vi "PDF_Interface_PDF Protokoll EPA1065_InterferenceVerification.vi"(8 "error in (no error)":errorcluster caption="Fehler (Eingang, kein Fehler)", 11 "Save PDF File Path":path) -> (0 "error out":errorcluster caption="Fehler (Ausgang)")   [LabVIEW 2020, in "EPA 1065.lvlib" / "Interference verificaton 1065-366.lvlib"]
uses:
  Interference verificaton 1065-366.lvlib
  Visualisierungs Elemente/String - Ausgabefeld.ctl
  ResultTable.ctl
  Sprachverwaltung/FGV Aktion Tabelle zerlegen.ctl
  <vilib>/Utility/miscctls.llb/LVRowAndColumnTypeDef.ctl
  Aktion FGV Interference.ctl
  Seiten/FT-IR/FGV FT-IR Aktionen.ctl
  Aktion Index uebersetzten.ctl
  Seiten/System Einstellungen V2/Aktioen FGV System Konstanten.ctl
  PDF_Interface/PDF Protokoll Standard Kopf Optionen.ctl
  <vilib>/Simplicity AI/SAI_PDF_API/Classes/Context/Controls/SAI_PDF_PDF Details.ctl
  PDF_Interface/PDF Interface Helper/PDFContentType.ctl
  PDF_Interface/PDF Interface Helper/PDFTableContentType.ctl
  PDF_Interface/PDF Interface Helper/PDFResults.ctl
  PDF_Interface/PDF Interface Helper/PDFResultPictures.ctl
  PDF_Interface/PDF Interface Helper/PDFCommentPosition.ctl
  PDF_Interface/PDF Interface Helper/PDFPageBreak.ctl
  PDF_Interface/PDF Interface Helper/PDFTablePictures.ctl
  PDF_Interface/PDF Interface Helper/PDFBemerkung.ctl
  <vilib>/Simplicity AI/SAI_PDF_API/Classes/Context/Controls/SAI_PDF_Text Align.ctl
  <vilib>/Simplicity AI/SAI_PDF_API/Classes/Context/Controls/SAI_PDF_Font.ctl
  <vilib>/Simplicity AI/SAI_PDF_API/Classes/Context/Controls/SAI_PDF_Font Encoding.ctl
  Allgemein/allgemeine Sub-VIs.lvlib
  Seiten/FT-IR/Span/Spanfaktor.lvlib
  Seiten/FT-IR/FT-IR.lvlib
  Sprachverwaltung/Sprachverwaltung.lvlib
  Seiten/System Einstellungen V2/System Einstellungen V2.lvlib
  PDF_Interface/PDF Interface.lvlib
  PDF_Interface/PDF Interface Helper/PDF Interface Helper.lvlib
  <vilib>/Simplicity AI/SAI_PDF_API/Classes/Context/Context.lvclass
  Linearisierung V2/Protokoll/Protokoll.lvlib
panel:
  out "Grenze in ppm:":sgl=2.0 caption="Limit in ppm:" min=0 format="%#.6g"
  out "[%]":sgl=2.0 caption="Limit:" min=0 format="%#.6g"
  out "LIN Ausgabetabelle":T1
  out "[%]":sgl=120.0 caption="Interference:" min=0 format="%#.6g"
  out "Konzentration Komponente":sgl=120.0 caption="Concentration:" min=0
  out "Komponente:":T2 caption="ppm"
  out "max. Flow Weighted Mean:":T2 caption="%"
  out "Konzentration FlowWeightedMean":sgl=120.0 caption="Concentration:" min=0 format="%#.2f"
  out "Ergebnis Tabelle":string[][](table) caption="Tabelle 3"
  out "Header Tabelle":string[][](table) caption="Tabelle"
  # "Interference Verification - EPA § 1065.366"
  # "Result"
  # "Analysis"
  # "Interference for Component:"
  # "Expected Flow weighted mean:"
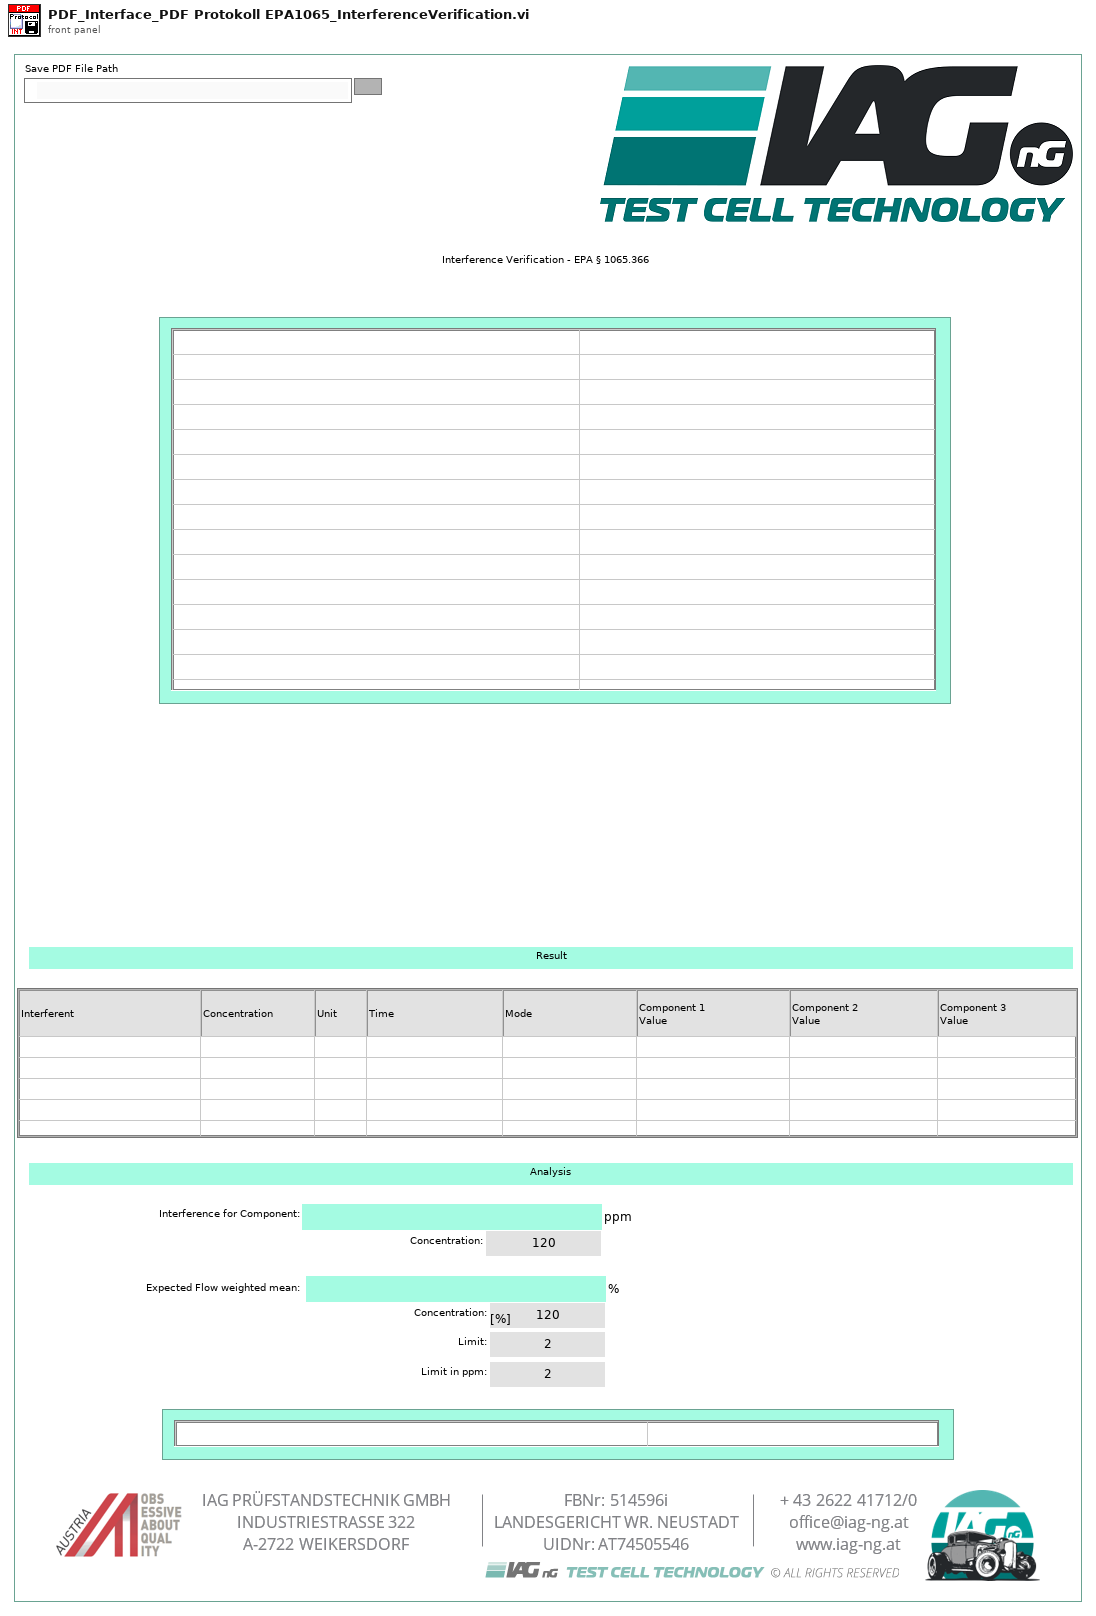
[diagram p1: front panel]
types:
  T1 = typedef "EPA 1065.lvlib/Interference verificaton 1065-366.lvlib/ResultTable.ctl" = string[][]
  T2 = typedef "String - Ausgabefeld.ctl" = string
  T3 = typedef "Sprachverwaltung.lvlib/FGV Aktion Tabelle zerlegen.ctl" = enum16{"laden", "vereinzeln", "speichern"}
  T4 = typedef "PDF Interface.lvlib/PDF Protokoll Standard Kopf Optionen.ctl" = cluster{"Analysator":bool, "FT-IR Rezept":bool, "Gasteiler":bool, "Gas Komponente":bool, "Gas Flasche":bool, "LIN Protokoll":bool, "Operator":bool}
  T5 = typedef "System Einstellungen V2.lvlib/Aktioen FGV System Konstanten.ctl" = enum16{"lesen", "laden", "speichern", "Sprache"}
  T6 = typedef "EPA 1065.lvlib/Interference verificaton 1065-366.lvlib/Aktion Index uebersetzten.ctl" = enum16{"lesen", "schreiben", "auswerten"}
  T7 = typedef "FT-IR.lvlib/FGV FT-IR Aktionen.ctl" = enum16{"lesen", "NOG setzen", "NOS setzen", "Initialisieren", "speichern", "ALLES setzen", "FT-IR Spektrum loggen", "Komm Stoppen", "Spektrum LogKonfig"}
  T8 = typedef "EPA 1065.lvlib/Interference verificaton 1065-366.lvlib/Aktion FGV Interference.ctl" = enum16{"Lesen", "TestKonfig", "TestSetting", "Einheiten", "Ergebnis", "Laden", "Tabelle", "Speichern", "löschen"}
  T9 = typedef "LVRowAndColumnTypeDef.ctl" = cluster{"Row":i32, "Column":i32}
  T10 = typedef "PDF Interface.lvlib/PDF Interface Helper.lvlib/PDFPageBreak.ctl" = enum16{"none", "before", "after", "after comment"}
  T11 = typedef "PDF Interface.lvlib/PDF Interface Helper.lvlib/PDFResults.ctl" = cluster{"Results":cluster{"Result Text":string, "Result":bool}[], "ResultPictures":T12, "use Pictures":bool, "Image Scale (%)":sgl, "Autoscale? (T)":bool, "Horizontal Align":i32, "Position":i32}
  T12 = typedef "PDF Interface.lvlib/PDF Interface Helper.lvlib/PDFResultPictures.ctl" = cluster{"Yes Ctl Refnum":refnum<vi>, "No Ctl Refnum":refnum<vi>}
  T13 = typedef "PDF Interface.lvlib/PDF Interface Helper.lvlib/PDFContentType.ctl" = cluster{"Titel":string, "Header Table":string[][], "Table Array":T14[], "Bemerkungen":T17[]}
  T14 = typedef "PDF Interface.lvlib/PDF Interface Helper.lvlib/PDFTableContentType.ctl" = cluster{"TableHeader":string[], "Table":string[][], "Relative Column Widths (%)":sgl[], "Results":T11, "PositionBemerkung":T15, "PageBreak":T10, "TablePictures":T16, "Horizontal Align":i32}
  T15 = typedef "PDF Interface.lvlib/PDF Interface Helper.lvlib/PDFCommentPosition.ctl" = enum16{"before", "after"}
  T16 = typedef "PDF Interface.lvlib/PDF Interface Helper.lvlib/PDFTablePictures.ctl" = cluster{"Ctl Refnum In":refnum<vi>[], "RowOrColumn":enum16{"Row", "Column"}, "IndexToInsert":u16, "Image Scale (%)":sgl[], "Autoscale? (T)":bool[], "Horizontal Align":i32}
  T17 = typedef "PDF Interface.lvlib/PDF Interface Helper.lvlib/PDFBemerkung.ctl" = cluster{"Bemerkung Text":string, "Align (Left)":T18, "Add Line Feeds (F:No)":bool, "Font":T19}
  T18 = typedef "SAI_PDF_Toolkit.lvlib/Context.lvclass/SAI_PDF_Text Align.ctl" = i32
  T19 = typedef "SAI_PDF_Toolkit.lvlib/Context.lvclass/SAI_PDF_Font.ctl" = cluster{"Font":string, "Size":i32, "Colour":u32, "Bold":bool, "Italic":bool, "Underline":bool, "Strikethrough":bool, "Font Encoding":T20}
  T20 = typedef "SAI_PDF_Toolkit.lvlib/Context.lvclass/SAI_PDF_Font Encoding.ctl" = enum16{"Cp1252, WinANSI", "IdentityH", "IdentityV", "Cp1250", "Cp1257", "MacRoman"}
  T21 = typedef "SAI_PDF_Toolkit.lvlib/Context.lvclass/SAI_PDF_PDF Details.ctl" = cluster{"Title":string, "Subject":string, "Keywords":string, "Author":string, "Creator":string}
  T22 = cluster{"Header Footer Text Cluster":cluster{"Header Text":string, "Footer Text":string, "Time":string, "Page Number":string}, "PDF Details":T21}
  T23 = typedef "EPA 1065.lvlib/Interference verificaton 1065-366.lvlib/TestSetting.ctl" = cluster{"Bearbeiter:":string, "Pfad:":path, "Textname:":string, "Analysator":T24}
  T24 = typedef "System Einstellungen V2.lvlib/Analysatoren.ctl" = string
  T25 = typedef "EPA 1065.lvlib/Interference verificaton 1065-366.lvlib/TestKonfig.ctl" = cluster{"CH4:":u16, "Ethane:":u16, "NMHC:":u16, "NMNEHC:":u16, "Komp 1 aktiv:":bool, "Komp 2 aktiv:":bool, "Komp 3 aktiv:":bool, "Komp 4 aktiv:":bool, "Modus":T26, "CG Aufschaltzeit:":dbl, "Interferent 1: CO2":u16, "Interferent 2: H2O":u16, "Interferent 3: CH4":u16, "Interferent 4: C2H6 / C3H8":u16, "Gasflaschen Nr.:":string, "Gasflaschen Nr.: 3":string, "Gasflaschen Nr.: 4":string, "Inter 1 aktiv":bool, "Inter 2 aktiv":bool, "Inter 3 aktiv":bool, "Inter 4 aktiv":bool, "Accuracy":string, "Accuracy 3":string, "Accuracy 4":string, "Konzentration 1:":dbl, "Konzentration 2:":dbl, "Konzentration 3:":dbl, "Konzentration 4:":dbl, "Flow weighted mean 1:":dbl, "Flow weighted mean 2:":dbl, "Flow weighted mean 3:":dbl, "Flow weighted mean 4:":dbl}
  T26 = typedef "EPA 1065.lvlib/Interference verificaton 1065-366.lvlib/Modus.ctl" = u16
  T27 = typedef "EPA 1065.lvlib/Interference verificaton 1065-366.lvlib/Komponenten.ctl" = cluster{"Komponente":T2, "Komponente Index":i32, "Komponente 2":T2, "Komponente Index 2":i32, "Komponente 3":T2, "Komponente Index 3":i32, "Komponente 4":T2, "Komponente Index 4":i32, "Interferent 1":T2, "Interferent Index":i32, "Interferent 2":T2, "Interferent 2 Index":i32, "Interferent 3":T2, "Interferent 3 Index":i32, "Interferent 4":T2, "Interferent 4 Index":i32}
  T28 = cluster{"Modell":string, "ProjektNummer":string, "Software Version":string, "Seriennummer":string}
  T29 = cluster{"Header Size":i32, "Column Ratio left":sgl[]}
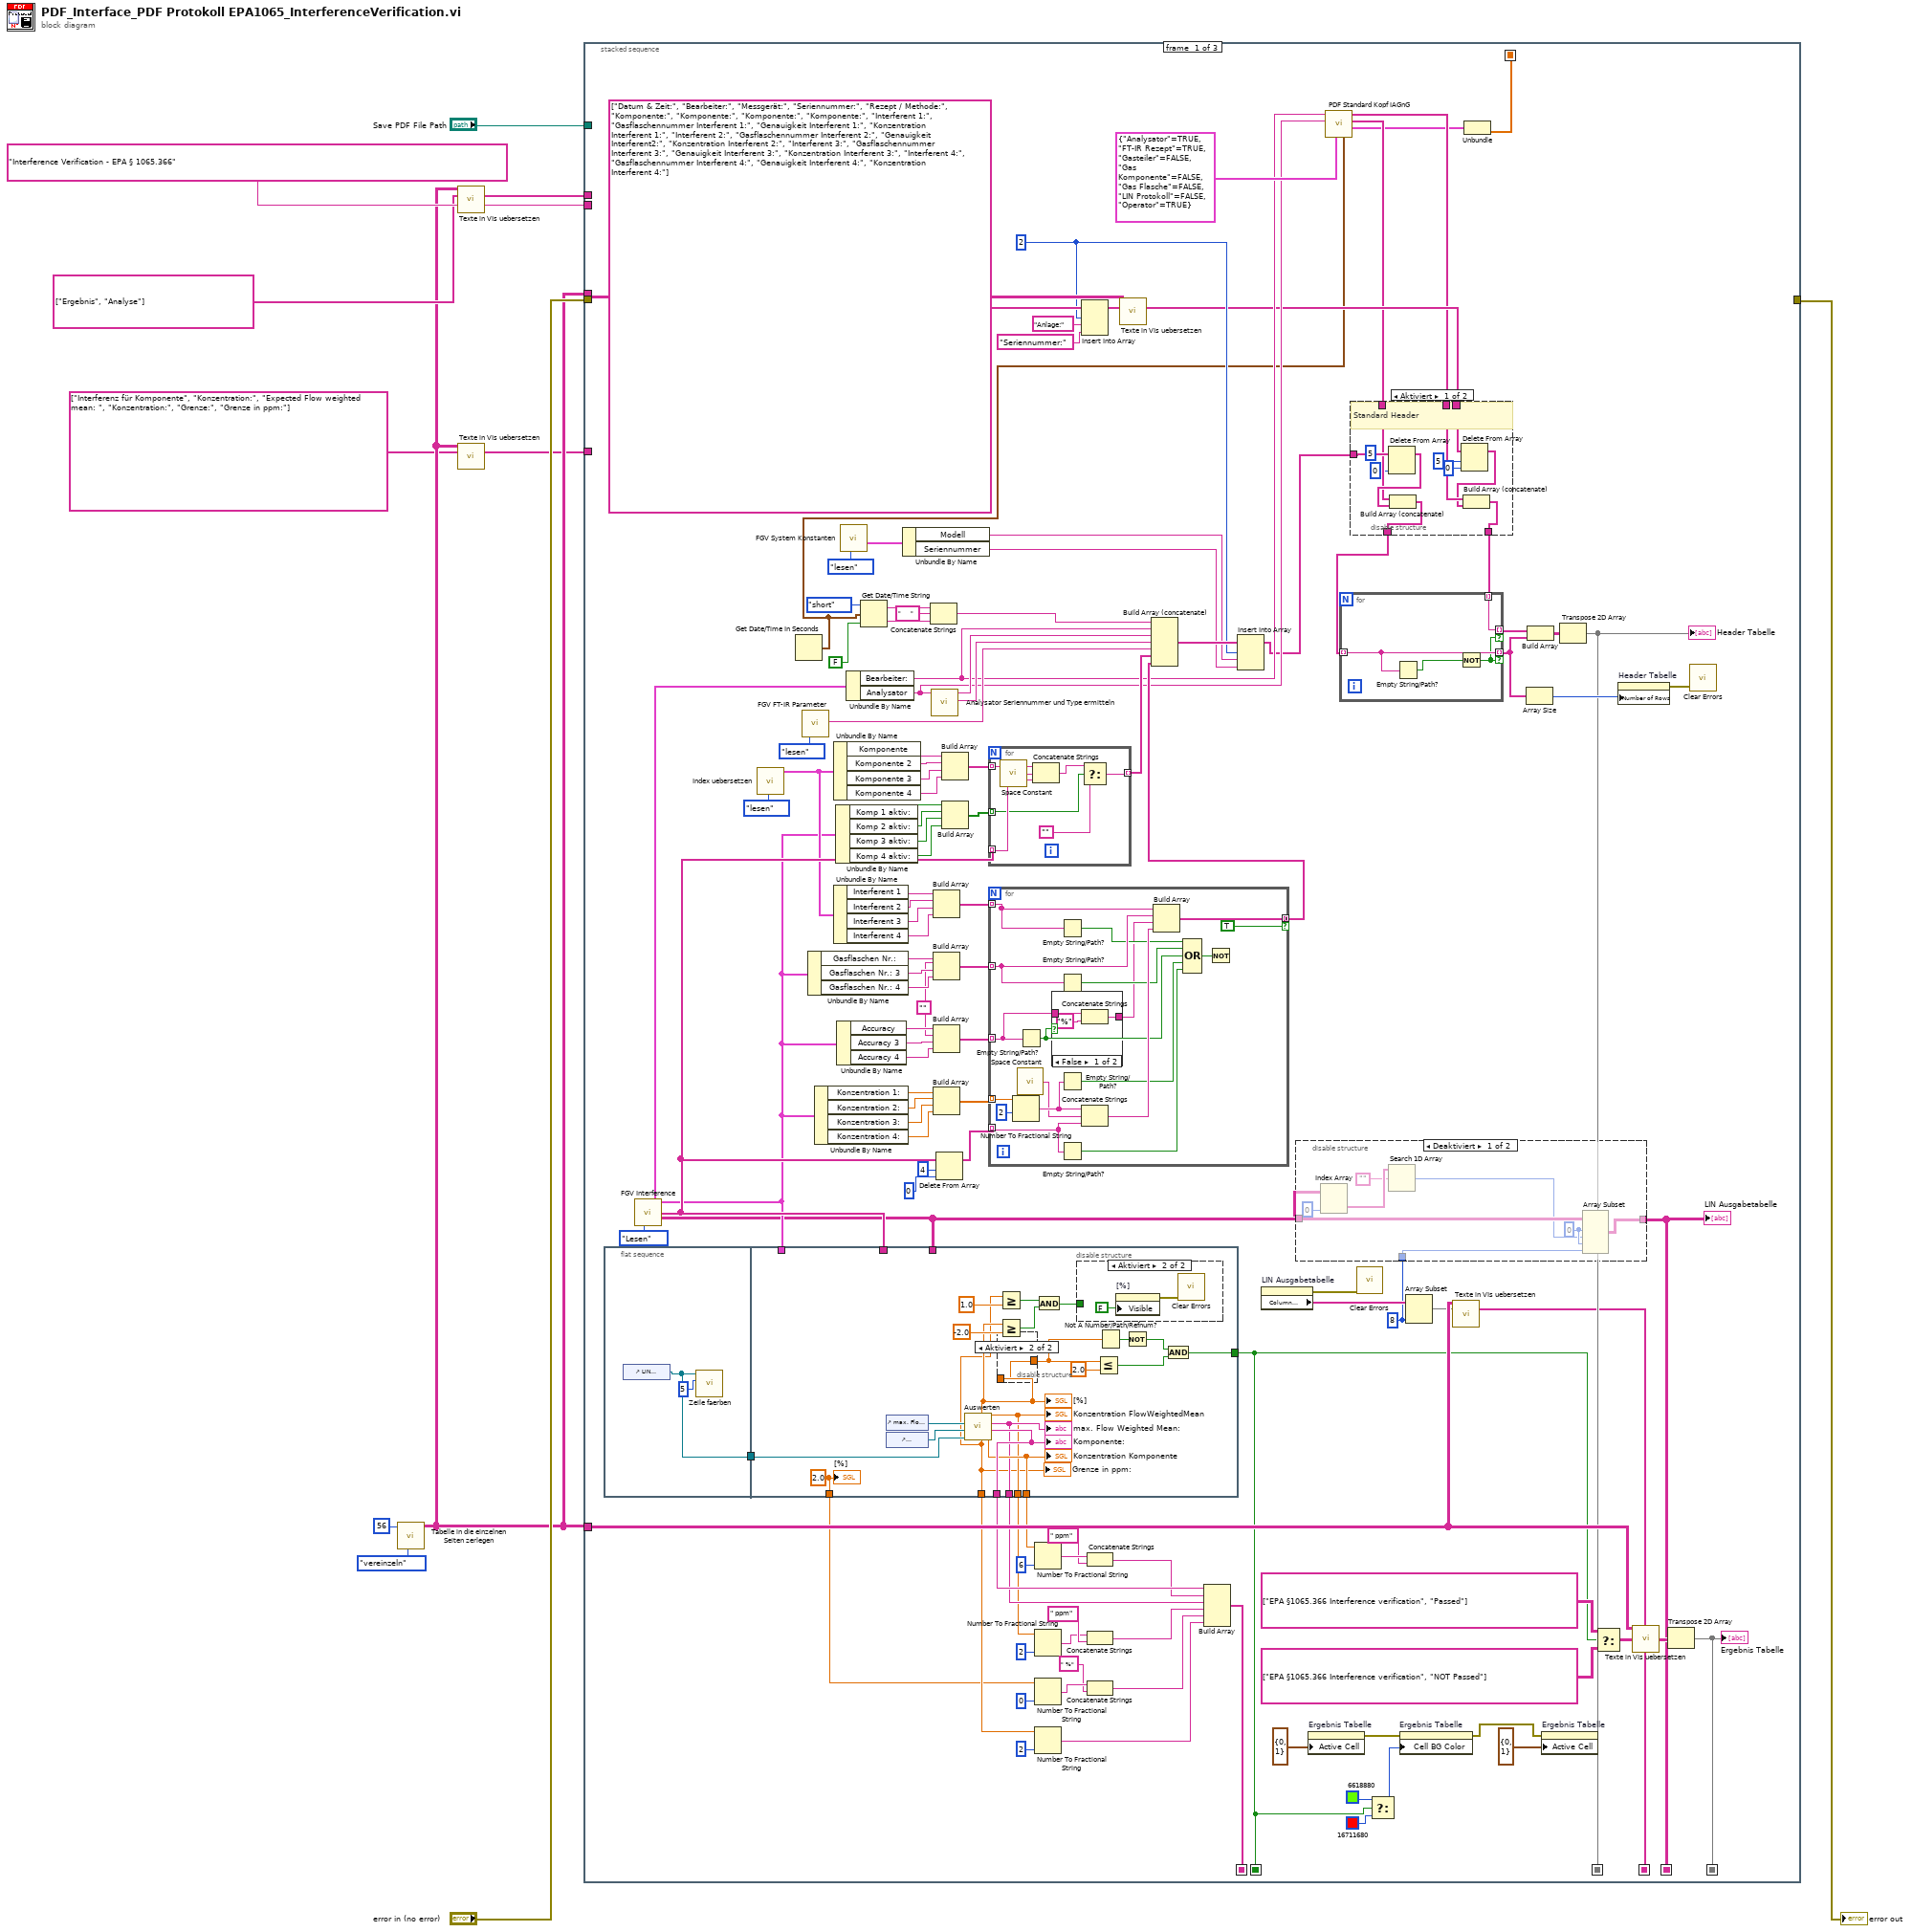
[diagram p0: block diagram]
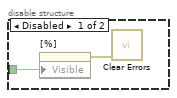
[diagram p5: hidden frame]
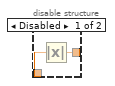
[diagram p6: hidden frame]
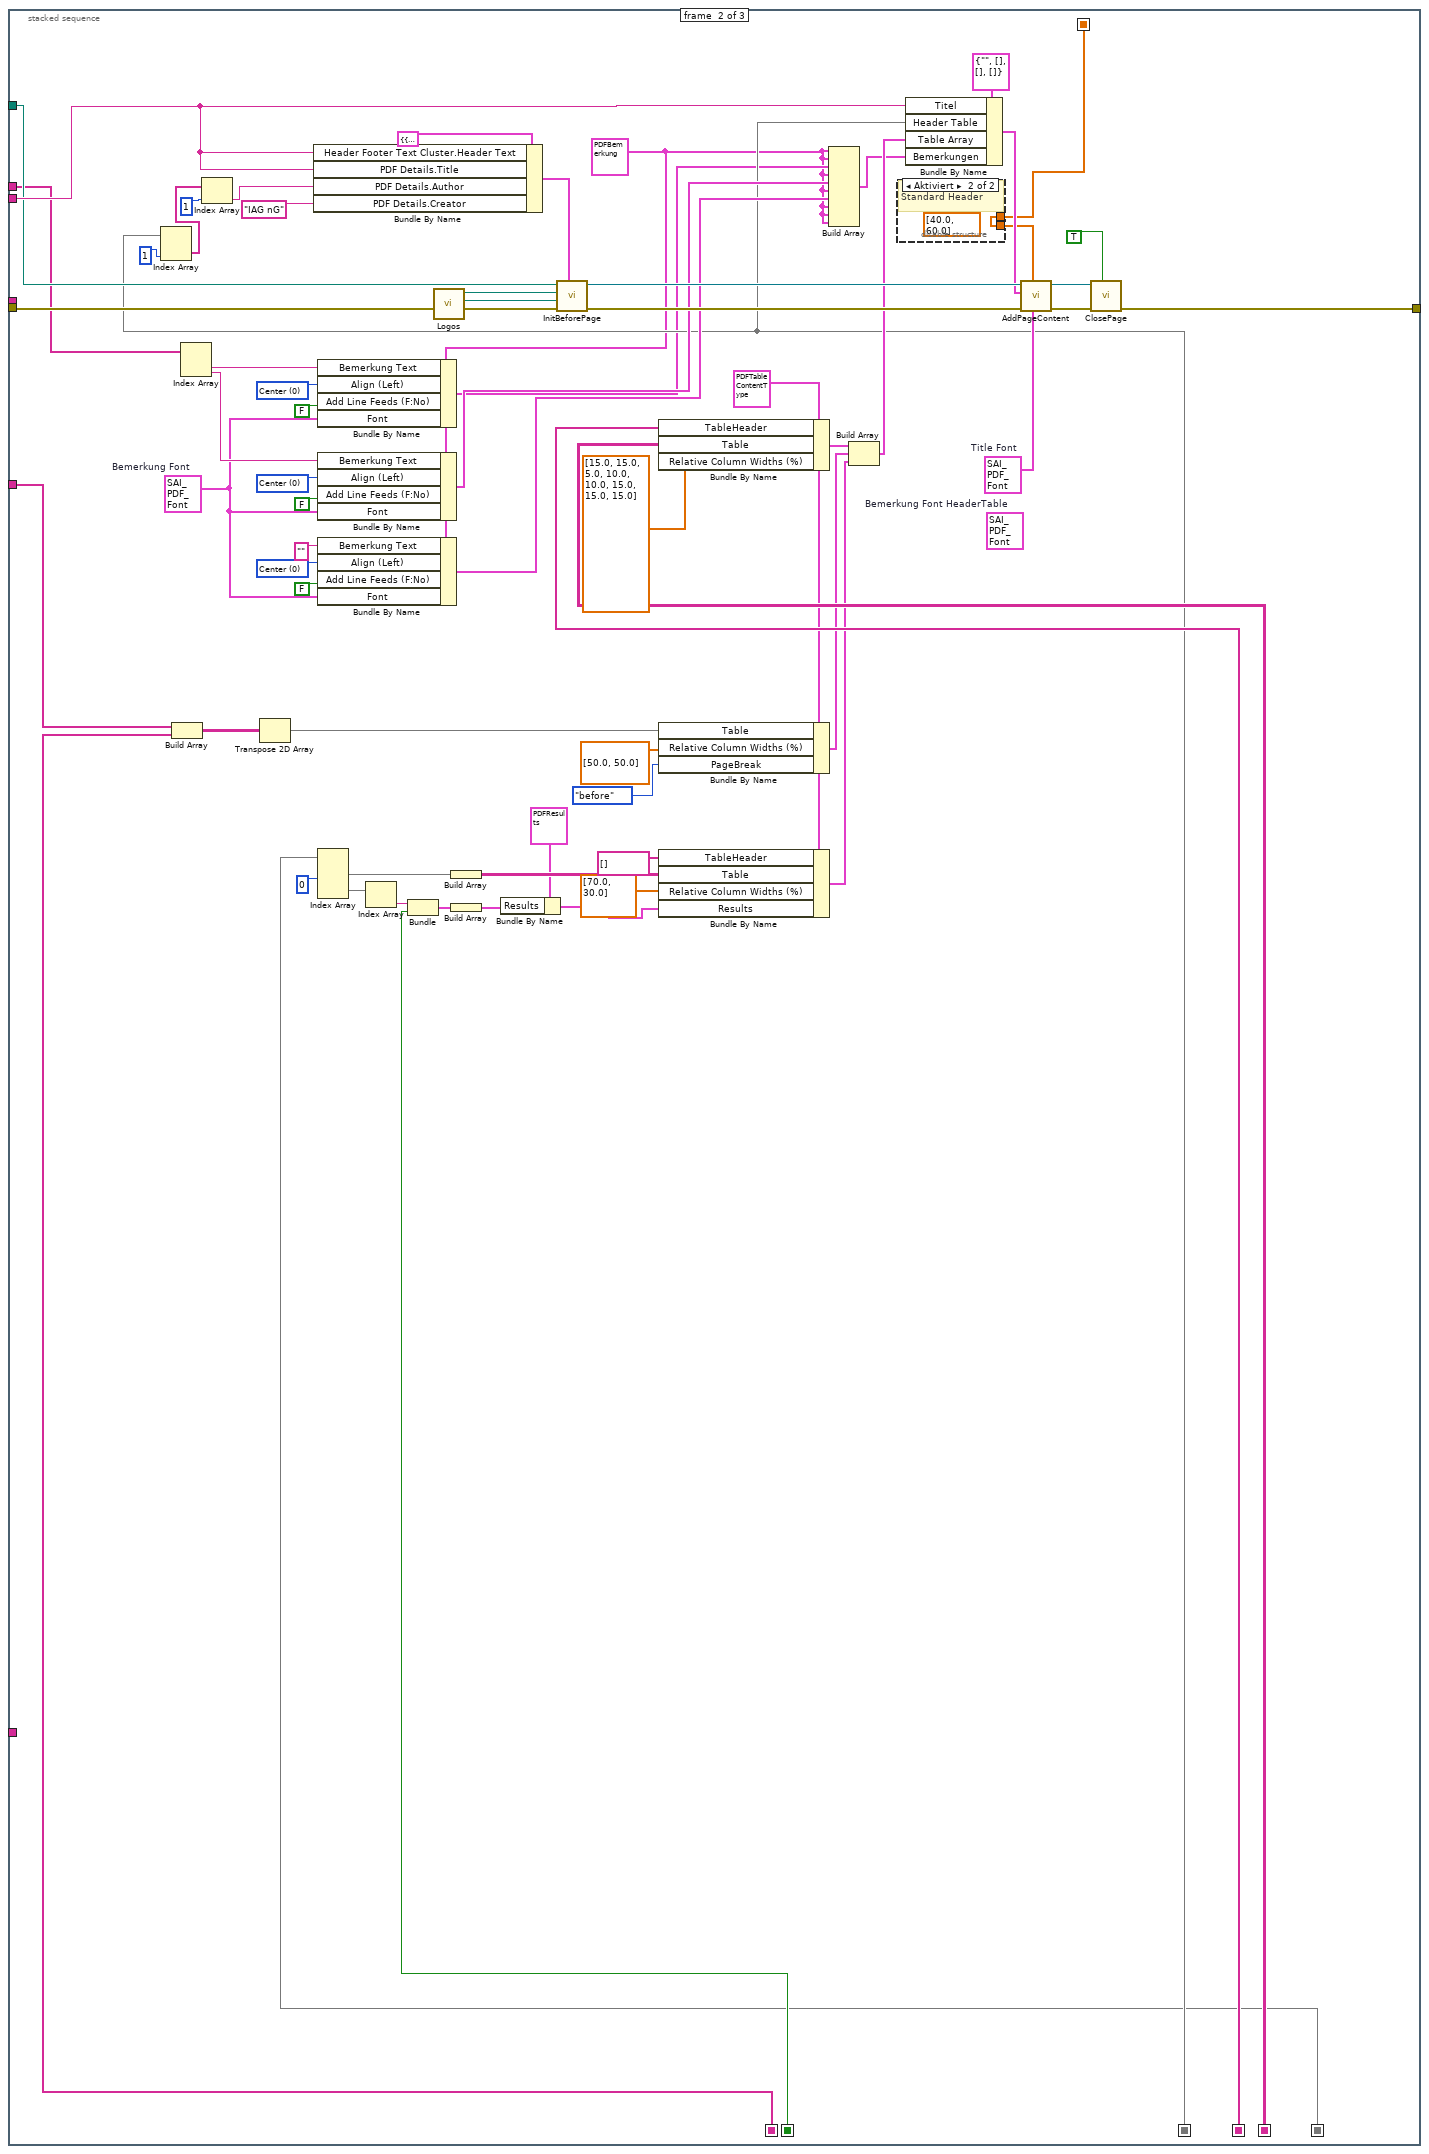
[diagram p7: hidden frame]
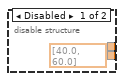
[diagram p8: hidden frame]
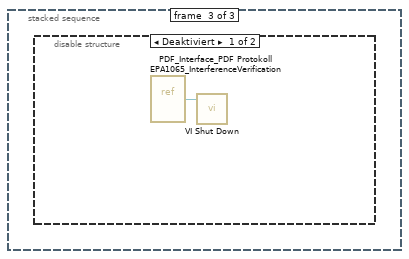
[diagram p9: hidden frame]
diagram:
  n1 = call "Tabelle in die einzelnen Seiten zerlegen.vi"("Aktion"=FGV_Aktion_Tabelle_zerlegen."vereinzeln", "Index (Seite)"=56) -> ("Sprachliste"=w3:string[][])  [unwired: 7 in, 2 out]
  n2 = call "Texte in VIs uebersetzen.vi"("Sprachliste"=w3, "String-Array zum Übersetzen"=string[] ["Ergebnis", "Analyse"], "String zum Übersetzen"="Interference Verification - EPA § 1065.366") -> ("String-Array zum Übersetzen"=w7:string[], "String zum Übersetzen"=w6:string)  [unwired: 8 in, 3 out]
  n3 = call "Texte in VIs uebersetzen.vi"("Sprachliste"=w3, "String-Array zum Übersetzen"=string[] ["Interferenz für Komponente", "Konzentration:", "Expected Flow weighted mean: ", "Konzentration:", "Grenze:", "Grenze in ppm:"]) -> ("String-Array zum Übersetzen"=w1:string[])  [unwired: 9 in, 4 out]
  n4 = stacked-sequence {
    seq-local: [w56 _ _] -> [_ w243 _]
    seq-local: [w55 _ _] -> [_ w244 _]
    seq-local: [w57 _ _] -> [_ w254 _]
    seq-local: [w37 _ _] -> [_ w249 _]
    seq-local: [w31 _ _] -> [_ w264 _]
    seq-local: [w36 _ _] -> [_ w265 _]
    seq-local: [w13 _ _] -> [_ w221 _]
    tunnel: w3 -> [w58 _ _]
    tunnel: w3 -> [w72 _ _]
    tunnel: "Save PDF File Path" -> [_ w268 _]
    tunnel: w7 -> [_ w255 _]
    tunnel: w6 -> [_ w269 _]
    tunnel: "error in (no error)" -> [_ w267 _]
    tunnel: [_ w266 _] -> w4
    tunnel: w1 -> [_ w230 _]
    frame #0 {
      w32 = 8 ("Länge")
      w61 = ""
      w62 = 2 ("Index")
      n5 = flat-sequence {
        tunnel: [w191] -> w125
        tunnel: w125 -> [w213]
        tunnel: [w205] -> w55
        tunnel: w99 -> [_]
        tunnel: w30 -> [_]
        tunnel: w71 -> [_]
        tunnel: [w198] -> w54
        tunnel: [w197] -> w53
        tunnel: [w196] -> w48
        tunnel: [w195] -> w46
        tunnel: [w194] -> w41
        tunnel: [w193] -> w38
        frame #0 {
          n6 = control-ref of="LIN Ausgabetabelle"() -> (w191:refnum<vi>)
          n7 = call "Zeile faerben.vi"("Anzahl"=5, "Table (Eingang)"=w191) -> ()  [unwired: 9 in, 1 out]
        }
        frame #1 {
          w193 = sgl 2.0 ("[%]")
          n8 = control-ref of="max. Flow Weighted Mean:"() -> (w212:refnum<vi>)
          n9 = control-ref of="Komponente:"() -> (w211:refnum<vi>)
          n10 = call "Auswerten.vi"("LIN Ausgabetabelle"=w213, "Komponente:"=w211, "max. Flow Weighted Mean:"=w212) -> ("Konzentration Komponente"=w197:dbl, "Komponente:"=w198:T2, "max. Flow Weighted Mean:"=w196:T2, "Konzentration FlowWeightedMean"=w195:dbl, "Limit in ppm"=w194:dbl, "[%]"=w200:dbl)  [unwired: 3 in]
          "max. Flow Weighted Mean:" <- w196
          "Konzentration FlowWeightedMean" <- w195
          "Konzentration Komponente" <- w197
          "Komponente:" <- w198
          "[%]" <- w200
          "Grenze in ppm:" <- w194
          n11 = disable-structure shown="Aktiviert" {
            disable-tunnel: w200 -> [w219 w220]
            disable-tunnel: [w218 w220] -> w209
            frame Disabled {
              n12 = Absolute Value(x=w219) -> (abs(x)=w218:dbl)
            }
            frame Enabled {
            }
          }
          n13 = Greater Or Equal?(x=w194, y=1.0) -> (x >= y?=w202:bool)
          n14 = Greater Or Equal?(x=w200, y=-2.0) -> (x >= y?=w201:bool)
          n15 = And(x=w202, y=w201) -> (x .and. y?=w199:bool)
          n16 = disable-structure shown="Aktiviert" {
            disable-tunnel: w199 -> [w215 _]
            frame Disabled {
              n17 = property on="[%]" class="DigWert (strikt)"("Visible"=w215) -> (error out=w214:errorcluster)  [unwired: 2 in, 1 out]
              n18 = call <vilib>:"Clear Errors.vi"("error in (no error)"=w214) -> ()  [unwired: 5 in, 2 out]
            }
            frame Enabled {
              n19 = property on="[%]" class="DigWert (strikt)"("Visible"=FALSE ("Sichtbar")) -> (error out=w217:errorcluster)  [unwired: 2 in, 1 out]
              n20 = call <vilib>:"Clear Errors.vi"("error in (no error)"=w217) -> ()  [unwired: 5 in, 2 out]
            }
          }
          n21 = Less Or Equal?(x=w209, y=2.0) -> (x <= y?=w207:bool)
          n22 = Not A Number/Path/Refnum?(number/path/refnum=w209) -> (NaN/Path/Refnum?=w208:bool)
          n23 = Not(x=w208) -> (.not. x?=w206:bool)
          n24 = And(x=w206, y=w207) -> (x .and. y?=w205:bool)
          "[%]" <- w193
        }
      }
      n25 = call "FGV Interference.vi"("Aktion FGV Interference"=Aktion_FGV_Interference."Lesen") -> ("TestSetting"=w123:T23, "TestKonfig"=w71:T25, "Êinheiten"=w99:string[], "Tabelle"=w30:T2[][])  [unwired: 9 in, 2 out]
      n26 = call "Index uebersetzen.vi"("Aktion"=Aktion_Index_uebersetzten."lesen") -> ("Komponenten"=w93:T27)  [unwired: 9 in, 1 out]
      n27 = Get Date/Time In Seconds() -> (seconds since 1Jan1904=w18:timestamp)
      n28 = call "FGV FT-IR Parameter.vi"("Aktion"=FGV_FT-IR_Aktionen."lesen") -> ("Current Recipe"=w105:string)  [unwired: 11 in, 7 out]
      n29 = Unbundle By Name(w71) -> ("Gasflaschen Nr.:"=w92:string, "Gasflaschen Nr.: 3"=w91:string, "Gasflaschen Nr.: 4"=w90:string)
      n30 = Unbundle By Name(w71) -> ("Konzentration 1:"=w89:dbl, "Konzentration 2:"=w88:dbl, "Konzentration 3:"=w87:dbl, "Konzentration 4:"=w86:dbl)
      n31 = Unbundle By Name(w93) -> ("Komponente"=w115:T2, "Komponente 2"=w114:T2, "Komponente 3"=w113:T2, "Komponente 4"=w60:T2)
      n32 = Unbundle By Name(w93) -> ("Interferent 1"=w97:T2, "Interferent 2"=w96:T2, "Interferent 3"=w95:T2, "Interferent 4"=w94:T2)
      n33 = Unbundle By Name(w71) -> ("Komp 1 aktiv:"=w112:bool, "Komp 2 aktiv:"=w111:bool, "Komp 3 aktiv:"=w110:bool, "Komp 4 aktiv:"=w59:bool)
      n34 = Unbundle By Name(w71) -> ("Accuracy"=w79:string, "Accuracy 3"=w78:string, "Accuracy 4"=w77:string)
      n35 = call "FGV System Konstanten.vi"("Aktionen"=Aktioen_FGV_System_Konstanten."lesen") -> ("Cluster out"=w69:T28)  [unwired: 6 in, 4 out]
      n36 = Unbundle By Name(w123) -> ("Bearbeiter:"=w26:string, "Analysator"=w25:T24)
      n37 = Get Date/Time String(date format (0)=enum16{"short", "long", "abbreviated"}."short" ("Datumsformat (0)"), seconds (now)=w18, want seconds? (F)=FALSE ("Angabe von Sekunden? (F)")) -> (date string=w122:string, time string=w121:string)
      n38 = Unbundle By Name(w69) -> ("Modell"=w66:string, "Seriennummer"=w65:string)
      n39 = Concatenate Strings(w122, "     " ("String"), w121) -> (w107:string)
      n40 = call "Analysator Seriennummer und Type ermitteln.vi"("Analysator"=w25) -> ("Type"=w28:string, "Name für Protokoll"=w29:string)  [unwired: 8 in, 1 out]
      n41 = Build Array(w97, w96, w95, w94) -> (w85:T2[])
      n42 = Build Array(w92, w61, w91, w90) -> (w84:string[])
      n43 = Build Array(w79, w61, w78, w77) -> (w76:string[])
      n44 = Build Array(w89, w88, w87, w86) -> (w83:dbl[])
      n45 = Delete From Array(array=w99, length=4 ("Länge"), index=0 ("Index")) -> (array with subset deleted=w81:string[])  [unwired: 1 out]
      n46 = Build Array(w115, w114, w113, w60) -> (w109:T2[])
      n47 = Build Array(w112, w111, w110, w59) -> (w108:bool[])
      n48 = for {
        tunnel: [w187] -> w106 mode=indexing
        tunnel: w109 -> [w190] mode=indexing
        tunnel: w108 -> [w186] mode=indexing
        tunnel: w99 -> [w189] mode=indexing
        n49 = call <vilib>:"Space Constant.vi"() -> ("String"=w188:string)
        n50 = Concatenate Strings(w190, w188, w189) -> (w185:string)
        n51 = Select(t=w185, s=w186, f="") -> (s? t:f=w187:string)
      }
      n52 = for {
        tunnel: w85 -> [w172] mode=indexing
        tunnel: w84 -> [w171] mode=indexing
        tunnel: w83 -> [w175] mode=indexing
        tunnel: w81 -> [w174] mode=indexing
        tunnel: [w169] -> w80 mode=concatenating if=TRUE
        tunnel: w76 -> [w159] mode=indexing
        n53 = Number To Fractional String(number=w175, precision (6)=i16 2 ("Genauigkeit (6)")) -> (F-format string=w173:string)  [unwired: 2 in]
        n54 = call <vilib>:"Space Constant.vi"() -> ("String"=w163:string)
        n55 = Empty String/Path?(string/path=w159) -> (empty?=w158:bool)
        n56 = case shown="False" w158 {
          tunnel: [w177 w179] -> w162
          tunnel: w159 -> [w176 w179]
          frame False {
            n57 = Concatenate Strings(w176, "%" ("String")) -> (w177:string)
          }
          frame True {
          }
        }
        n58 = Empty String/Path?(string/path=w172) -> (empty?=w168:bool)
        n59 = Empty String/Path?(string/path=w171) -> (empty?=w167:bool)
        n60 = Empty String/Path?(string/path=w173) -> (empty?=w164:bool)
        n61 = Empty String/Path?(string/path=w174) -> (empty?=w166:bool)
        n62 = Concatenate Strings(w173, w163, w174) -> (w170:string)
        n63 = Build Array(w172, w171, w162, w170) -> (w169:T2[])
        n64 = Compound Arithmetic op=OR ("Mehrfacharithmetik")(w168, w167, w158, w164, w166) -> (w165:bool)
        n65 = Not(x=w165) -> ()  [unwired: 1 out]
      }
      n66 = Number To Fractional String(number=w53, precision (6)=i16 6 ("Genauigkeit (6)")) -> (F-format string=w51:string)  [unwired: 2 in]
      n67 = Number To Fractional String(number=w46, precision (6)=i16 2 ("Genauigkeit (6)")) -> (F-format string=w44:string)  [unwired: 2 in]
      n68 = Number To Fractional String(number=w38, precision (6)=i16 0 ("Genauigkeit (6)")) -> (F-format string=w17:string)  [unwired: 2 in]
      n69 = Number To Fractional String(number=w41, precision (6)=i16 2 ("Genauigkeit (6)")) -> (F-format string=w40:string)  [unwired: 2 in]
      n70 = Insert Into Array(array=string[] ["Datum & Zeit:", "Bearbeiter:", "Messgerät:", "Seriennummer:", "Rezept / Methode:", "Komponente:", "Komponente:", "Komponente:", "Komponente:", "Interferent 1:", "Gasflaschennummer Interferent 1:", "Genauigkeit Interferent 1:", "Konzentration Interferent 1:", "Interferent 2:", "Gasflaschennummer Interferent 2:", "Genauigkeit Interferent2:", "Konzentration Interferent 2:", "Interferent 3:", "Gasflaschennummer Interferent 3:", "Genauigkeit Interferent 3:", "Konzentration Interferent 3:", "Interferent 4:", "Gasflaschennummer Interferent 4:", "Genauigkeit Interferent 4:", "Konzentration Interferent 4:"], index=w62, new element #1="Anlage:" ("Neues Element/Teil-Array"), new element #2="Seriennummer:" ("Neues Element/Teil-Array")) -> (w68:string[])
      n71 = Concatenate Strings(w51, " ppm" ("String")) -> (w49:string)
      n72 = Concatenate Strings(w44, " ppm" ("String")) -> (w43:string)
      n73 = Concatenate Strings(w17, " %" ("String")) -> (w15:string)
      n74 = call "Texte in VIs uebersetzen.vi"("Sprachliste"=w72, "String-Array zum Übersetzen"=w68) -> ("String-Array zum Übersetzen"=w23:string[])  [unwired: 9 in, 4 out]
      n75 = Build Array (concatenate)(w107, w26, w29, w28, w105, w106, w80) -> (w67:T2[])
      n76 = Build Array(w54, w49, w48, w43, w15, w40) -> (w37:T2[])
      n77 = Insert Into Array(array=w67, index=w62, new element #1=w66, new element #2=w65) -> (w21:T2[])
      n78 = property on="LIN Ausgabetabelle" class="Tbl (strikt)"() -> (error out=w33:errorcluster, "Column Headers[]"=w35:string[])  [unwired: 2 in, 1 out]
      n79 = disable-structure shown="Deaktiviert" {
        disable-tunnel: w32 -> [w141 _]
        disable-tunnel: [w140 w143] -> w31
        disable-tunnel: w30 -> [w139 w143]
        frame Disabled {
          w142 = 0 ("Index")
          n80 = Index Array(array=w139, index (col)=0 ("Deaktivierter Index (Spalte)")) -> (element=w137:T2[])  [unwired: 1 in]
          n81 = Search 1D Array(1D array=w137, element="") -> (index of element=w135:i32)  [unwired: 1 in]
          n82 = Array Subset(array=w139, index (row)=w142, length (row)=w135, index (col)=w142, length (col)=w141) -> (w140:T2[][])
        }
        frame Enabled {
        }
      }
      "LIN Ausgabetabelle" <- w31
      n83 = property on="Ergebnis Tabelle" class="Tbl (strikt)"("Active Cell"=T9 {"Row"=0, "Column"=1} ("Aktive Zelle:Aktive Zelle")) -> (error out=w130:errorcluster)  [unwired: 2 in, 1 out]
      n84 = call "PDF Standard Kopf IAGnG.vi"("Zeitstempel"=w18, "Oprtionen Cluster"=T4 {"Analysator"=TRUE, "FT-IR Rezept"=TRUE, "Gasteiler"=FALSE, "Gas Komponente"=FALSE, "Gas Flasche"=FALSE, "LIN Protokoll"=FALSE, "Operator"=TRUE}, "Analysator"=w25, "Bearbeiter/in"=w26) -> ("Size Cluster"=w14:T29, "Header Values"=w19:T2[], "Header Labels"=w22:string[])  [unwired: 4 in, 1 out]
      n85 = disable-structure shown="Aktiviert" {
        disable-tunnel: [w153 w157] -> w24
        disable-tunnel: w23 -> [w155 w157]
        disable-tunnel: w22 -> [w154 _]
        disable-tunnel: w21 -> [w149 w156]
        disable-tunnel: [w146 w156] -> w20
        disable-tunnel: w19 -> [w147 _]
        frame Enabled {
          # "Standard Header"
          n86 = Delete From Array(array=w149, length=5 ("Länge"), index=0 ("Index")) -> (array with subset deleted=w148:T2[])  [unwired: 1 out]
          n87 = Build Array (concatenate)(w147, w148) -> (w146:T2[])
          n88 = Delete From Array(array=w155, length=5 ("Länge"), index=0 ("Index")) -> (array with subset deleted=w152:string[])  [unwired: 1 out]
          n89 = Build Array (concatenate)(w154, w152) -> (w153:string[])
        }
        frame Disabled {
        }
      }
      n90 = for {
        tunnel: w20 -> [w183] mode=indexing
        tunnel: [w183] -> w102 mode=indexing if=w180
        tunnel: [w181] -> w104 mode=indexing if=w180
        tunnel: w24 -> [w181] mode=indexing
        n91 = Empty String/Path?(string/path=w183) -> (empty?=w182:bool)
        n92 = Not(x=w182) -> (.not. x?=w180:bool)
      }
      n93 = call <vilib>:"Clear Errors.vi"("error in (no error)"=w33) -> ()  [unwired: 5 in, 2 out]
      n94 = Select(t=u32 6618880, s=w55, f=u32 16711680) -> (s? t:f=w131:u32)
      n95 = property on="Ergebnis Tabelle" class="Tbl (strikt)"(error in=w130, "Cell BG Color"=w131) -> (error out=w126:errorcluster)  [unwired: 1 in, 1 out]
      n96 = Array Subset(array=w35, length=w32) -> (w34:string[])  [unwired: 1 in]
      n97 = call "Texte in VIs uebersetzen.vi"("Sprachliste"=w58, "String-Array zum Übersetzen"=w34) -> ("String-Array zum Übersetzen"=w36:string[])  [unwired: 9 in, 4 out]
      n98 = Unbundle(w14) -> ("Column Ratio left"=w13:sgl[])  [unwired: 1 out]
      n99 = Array Size(array=w102) -> (size(s)=w101:i32)
      n100 = Build Array(w104, w102) -> (w103:T2[][])
      n101 = property on="Ergebnis Tabelle" class="Tbl (strikt)"(error in=w126, "Active Cell"=T9 {"Row"=0, "Column"=1} ("Aktive Zelle:Aktive Zelle")) -> ()  [unwired: 1 in, 2 out]
      n102 = Transpose 2D Array(2D array=w103) -> (transposed array=w57:T2[][])
      "Header Tabelle" <- w57
      n103 = Select(t=string[][] [["EPA §1065.366 Interference verification"], ["Passed"]] ("Tabelle 3"), s=w55, f=string[][] [["EPA §1065.366 Interference verification"], ["NOT Passed"]] ("Tabelle 3")) -> (s? t:f=w75:string[][])
      n104 = property on="Header Tabelle" class="Tbl (strikt)"("Number of Rows"=w101) -> (error out=w100:errorcluster)  [unwired: 2 in, 1 out]
      n105 = call "Texte in VIs uebersetzen.vi"("Sprachliste"=w58, "2D String-Array zum Übersetzen"=w75) -> ("2D String-Array zum Übersetzen"=w74:string[][])  [unwired: 9 in, 4 out]
      n106 = Transpose 2D Array(2D array=w74) -> (transposed array=w56:string[][])
      "Ergebnis Tabelle" <- w56
      n107 = call <vilib>:"Clear Errors.vi"("error in (no error)"=w100) -> ()  [unwired: 5 in, 2 out]
    }
    frame #1 {
      w223 = T19 {"Font"="Arial", "Size"=12, "Colour"=0, "Bold"=TRUE, "Italic"=TRUE, "Underline"=FALSE, "Strikethrough"=FALSE, "Font Encoding"=enum."Cp1252, WinANSI"}  # Bemerkung Font
      w224 = T17 {"Bemerkung Text"="", "Align (Left)"=0, "Add Line Feeds (F:No)"=FALSE, "Font"={"Font"="Arial", "Size"=10, "Colour"=0, "Bold"=FALSE, "Italic"=FALSE, "Underline"=FALSE, "Strikethrough"=FALSE, "Font Encoding"=enum."Cp1252, WinANSI"}} ("Bemerkung")
      w228 = T14 {"TableHeader"=[], "Table"=[], "Relative Column Widths (%)"=[], "Results"={"Results"=[], "ResultPictures"={"Yes Ctl Refnum"=refnum, "No Ctl Refnum"=refnum}, "use Pictures"=FALSE, "Image Scale (%)"=0.0, "Autoscale? (T)"=FALSE, "Horizontal Align"=0, "Position"=0}, "PositionBemerkung"=enum."before", "PageBreak"=enum."none", "TablePictures"={"Ctl Refnum In"=[], "RowOrColumn"=enum."Row", "IndexToInsert"=0, "Image Scale (%)"=[], "Autoscale? (T)"=[], "Horizontal Align"=0}, "Horizontal Align"=0} ("Table Array")
      w233 = T18 0 items=["Center", "Justified", "Justified All", "Left", "Right"] ("Align (Left)")
      w258 = T18 0 items=["Center", "Justified", "Justified All", "Left", "Right"] ("Align (Left)")
      w261 = T18 0 items=["Center", "Justified", "Justified All", "Left", "Right"] ("Align (Left)")
      (unwired) T19 {"Font"="Arial", "Size"=12, "Colour"=16711680, "Bold"=TRUE, "Italic"=TRUE, "Underline"=FALSE, "Strikethrough"=FALSE, "Font Encoding"=enum."Cp1252, WinANSI"}  # Bemerkung Font HeaderTable
      w273 = T19 {"Font"="Arial", "Size"=24, "Colour"=0, "Bold"=TRUE, "Italic"=FALSE, "Underline"=TRUE, "Strikethrough"=FALSE, "Font Encoding"=enum."Cp1252, WinANSI"}  # Title Font
      n108 = Index Array(array=w254, index (col)=1 ("Index")) -> (element=w252:T2[])  [unwired: 1 in]
      n109 = Build Array(w230, w249) -> (w248:T2[][])
      n110 = Index Array(array=w255) -> (element #1=w231:string, element #2=w235:string)  [unwired: 2 in]
      n111 = Index Array(array=w252, index=1 ("Index")) -> (element=w270:T2)
      n112 = Transpose 2D Array(2D array=w248) -> (transposed array=w236:T2[][])
      n113 = Bundle By Name(cluster=T22 {"Header Footer Text Cluster"={"Header Text"="Protokoll XYZ", "Footer Text"="IAG nG", "Time"="<TIMESTAMP yyyy-MM-dd>", "Page Number"="Page <P> of <PT>"}, "PDF Details"={"Title"="Test PDF", "Subject"="Versa Tabasco", "Keywords"="", "Author"="RIW", "Creator"="IAG"}} ("Info"), "Header Footer Text Cluster.Header Text"=w269, "PDF Details.Title"=w269, "PDF Details.Author"=w270, "PDF Details.Creator"="IAG nG") -> (w278:T22)
      n114 = Bundle By Name(cluster=w224, "Bemerkung Text"=w231, "Align (Left)"=w233, "Add Line Feeds (F:No)"=FALSE, "Font"=w223) -> (w232:T17)
      n115 = Bundle By Name(cluster=w224, "Bemerkung Text"=w235, "Align (Left)"=w261, "Add Line Feeds (F:No)"=FALSE, "Font"=w223) -> (w257:T17)
      n116 = Bundle By Name(cluster=w224, "Bemerkung Text"="", "Align (Left)"=w258, "Add Line Feeds (F:No)"=FALSE, "Font"=w223) -> (w256:T17)
      n117 = Index Array(array=w243, index (col) #1=0 ("Deaktivierter Index (Spalte)")) -> (element #1=w238:string[], element #2=w241:string[])  [unwired: 3 in]
      n118 = Index Array(array=w241) -> (element=w240:string)  [unwired: 1 in]
      n119 = Bundle(w240, w244) -> (w239:cluster{string, bool})  [unwired: 1 in]
      n120 = call "Logos.vi"() -> ("Footer Image File Path"=w286:path, "Header Image File Path"=w287:path)  [unwired: 8 in, 2 out]
      n121 = Build Array(w238) -> (w237:string[][])
      n122 = Build Array(w239) -> (w227:cluster{string, bool}[])
      n123 = Bundle By Name(cluster=T11 {"Results"=[], "ResultPictures"={"Yes Ctl Refnum"=refnum, "No Ctl Refnum"=refnum}, "use Pictures"=FALSE, "Image Scale (%)"=100.0, "Autoscale? (T)"=TRUE, "Horizontal Align"=3, "Position"=0} ("Results"), "Results"=w227) -> (w226:T11)
      n124 = call "InitBeforePage.vi"("Info"=w278, "Fehler (Eingang, kein Fehler)"=w267, "Footer Image File Path"=w286, "Header Image File Path"=w287, "Path (Dialog if Empty)"=w268) -> ("Fehler (Ausgang)"=w285:errorcluster, "Context (Ausgang)"=w284:refnum<class "Context.lvclass">)  [unwired: 5 in]
      n125 = Bundle By Name(cluster=w228, "TableHeader"=w265, "Table"=w264, "Relative Column Widths (%)"=sgl[] [15.0, 15.0, 5.0, 10.0, 10.0, 15.0, 15.0, 15.0]) -> (w272:T14)
      n126 = Bundle By Name(cluster=w228, "Table"=w236, "Relative Column Widths (%)"=sgl[] [50.0, 50.0], "PageBreak"=PDFPageBreak."before") -> (w250:T14)
      n127 = Bundle By Name(cluster=w228, "TableHeader"=string[] [], "Table"=w237, "Relative Column Widths (%)"=sgl[] [70.0, 30.0], "Results"=w226) -> (w251:T14)
      n128 = Build Array(w224, w224, w232, w224, w257, w224, w256, w224, w224, w224) -> (w262:T17[])
      n129 = Build Array(w272, w250, w251) -> (w276:T14[])
      n130 = disable-structure shown="Aktiviert" {
        disable-tunnel: [sgl[] [40.0, 60.0] ("Column Ratio left") w289] -> w274
        disable-tunnel: w221 -> [_ w289]
        frame Disabled {
        }
        frame Enabled {
          (unwired) sgl[] [40.0, 60.0] ("Column Ratio left")
          # "Standard Header"
        }
      }
      n131 = Bundle By Name(cluster=T13 {"Titel"="", "Header Table"=[], "Table Array"=[], "Bemerkungen"=[]} ("Content"), "Titel"=w269, "Header Table"=w254, "Table Array"=w276, "Bemerkungen"=w262) -> (w275:T13)
      n132 = call "AddPageContent.vi"("Title Font"=w273, "Column Ratio left"=w274, "error in"=w285, "Content"=w275, "Context (Eingang)"=w284) -> ("error out"=w283:errorcluster, "Context (Ausgang)"=w282:refnum<class "Context.lvclass">)  [unwired: 5 in]
      n133 = call "ClosePage.vi"("popup viewer"=TRUE, "Fehler (Eingang, kein Fehler)"=w283, "Context (Eingang)"=w282) -> ("Fehler (Ausgang)"=w266:errorcluster)  [unwired: 8 in]
    }
    frame #2 {
      n134 = disable-structure shown="Deaktiviert" {
        frame Disabled {
          n135 = vi-ref "PDF_Interface_PDF Protokoll EPA1065_InterferenceVerification.vi"() -> (w290:refnum<vi>)
          n136 = call "VI Shut Down.vi"("VI Referenz"=w290) -> ()  [unwired: 11 in]
        }
        frame Enabled {
        }
      }
    }
  }
  "error out" <- w4
